vi "Returning A Value Complex Struct Added.vi"(8 "error in (no error)":errorcluster) -> ()   [LabVIEW 2009, in "LabVIEWWrapper_PassingDataSampleDLL.lvlib"]
doc: "int ReturningAValue_Integer (void);"
uses:
  LabVIEWWrapper_PassingDataSampleDLL.lvlib
  CustomControlsForStructs/ComplexStruct Polygon.ctl
  <vilib>/Utility/importsl/GetValueByPointer/GetValueByPointer.xnode
  <vilib>/Utility/importsl/GetValueByPointer/datatype.ctl
  PassingDataSampleDLL.dll
  Program Files (x86)/National Instruments/LabVIEW 2009/resource/lvimptsl.dll
panel:
  out "ComplexStruct Polygon":T1
  out "error out":errorcluster
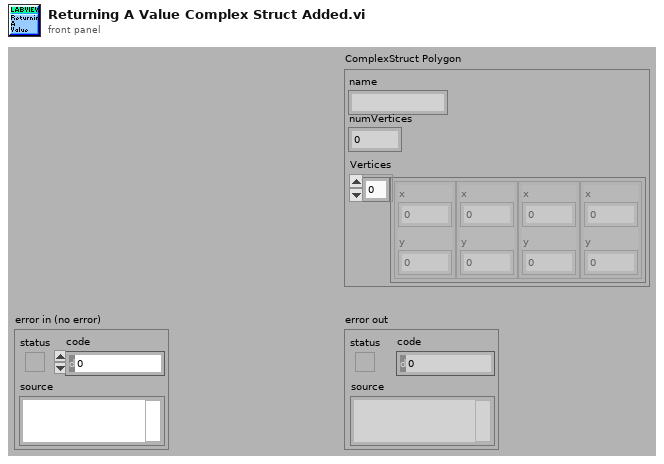
[diagram p1: front panel]
types:
  T1 = typedef "LabVIEWWrapper_PassingDataSampleDLL.lvlib/ComplexStruct Polygon.ctl" = cluster{"name":string, "numVertices":i32, "Vertices":cluster{"x":i32, "y":i32}[]}
  T2 = cluster{"Output":string, "Destination":i32, cluster{"Output":i32, "Output":i32}[]}
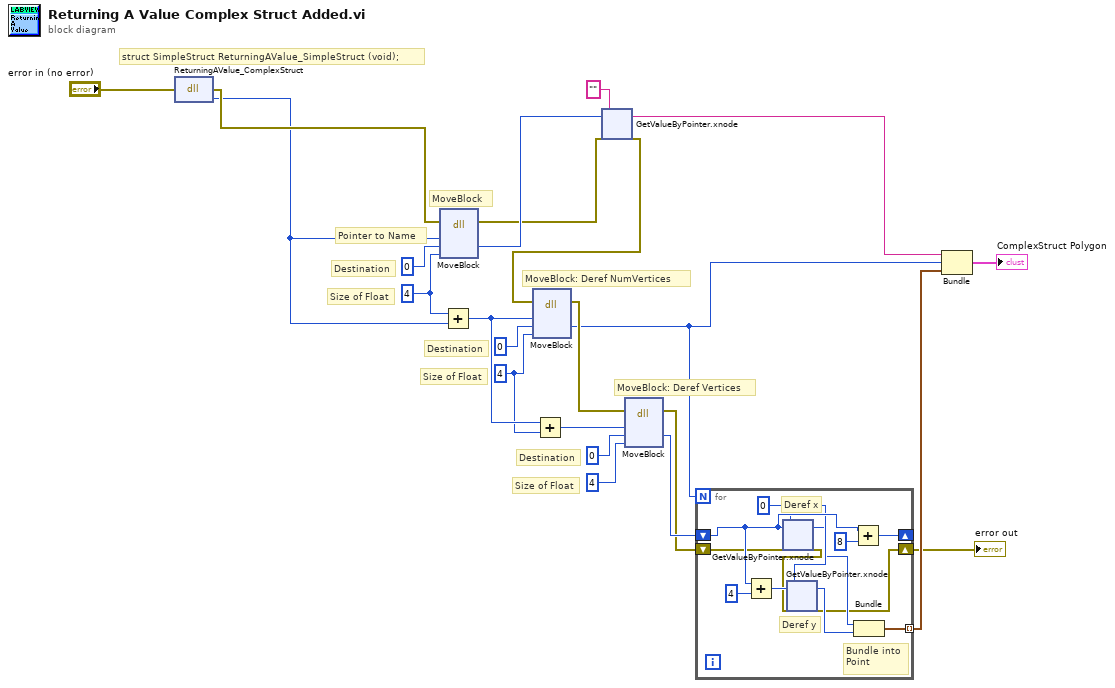
[diagram p0: block diagram]
diagram:
  w16 = 4 ("arg3")
  w14 = 4 ("arg3")
  # "Pointer to Name"
  # "Destination"
  # "Size of Float"
  # "MoveBlock: Deref Vertices"
  # "Destination"
  # "Size of Float"
  # "MoveBlock: Deref NumVertices"
  # "Destination"
  # "Size of Float"
  # "MoveBlock"
  # "struct SimpleStruct ReturningAValue_SimpleStruct (void);"
  n1 = dll-call lib="C:/My Dropbox/Systems Engineering Application/SDK/C Integration/LabVIEWWrapper/PassingDataSampleDLL.*" fn="ReturningAValue_ComplexStruct"(error in="error in (no error)") -> (error out=w8:errorcluster, "return type"=w7:i32)  [unwired: 2 in, 1 out]
  n2 = dll-call lib="LabVIEW" fn="MoveBlock"(error in=w8, "Address (Pointer)"=w7, "Destination"=0, "Size"=w14) -> (error out=w10:errorcluster, "Destination"=w12:i32)  [unwired: 5 in, 1 out]
  n3 = Add(x=w14, y=w7) -> (x+y=w17:i32)
  n4 = Add(x=w17, y=w16) -> (x+y=w18:i32)
  n5 = xnode "GetValueByPointer.xnode"("Pointer"=w12, "InputType"="", "ErrorIn"=w10) -> ("Output"=w5:string, "ErrorOut"=w9:errorcluster)  [unwired: 1 in]
  n6 = dll-call lib="LabVIEW" fn="MoveBlock"(error in=w9, "Address (Pointer)"=w17, "Destination"=0, "Size"=w16) -> (error out=w11:errorcluster, "Destination"=w4:i32)  [unwired: 5 in, 1 out]
  n7 = dll-call lib="LabVIEW" fn="MoveBlock"(error in=w11, "Address (Pointer)"=w18, "Destination"=0, "Size"=4 ("arg3")) -> (error out=w2:errorcluster, "Destination"=w15:i32)  [unwired: 5 in, 1 out]
  n8 = for {
    N: w4 -> [_]
    shift-right: [w31] -> _
    shift-left: w15 -> [w32]
    tunnel: [w27] -> w3 mode=indexing
    shift-right: [w24] -> w1
    shift-left: w2 -> [w26]
    w30 = 0
    # "Deref y"
    # "Deref x"
    # "Bundle into\nPoint"
    n9 = Add(x=w32, y=4) -> (x+y=w35:i32)
    n10 = xnode "GetValueByPointer.xnode"("Pointer"=w32, "InputType"=w30, "ErrorIn"=w26) -> ("Output"=w29:i32, "ErrorOut"=w25:errorcluster)  [unwired: 1 in]
    n11 = xnode "GetValueByPointer.xnode"("Pointer"=w35, "InputType"=w30, "ErrorIn"=w25) -> ("Output"=w28:i32, "ErrorOut"=w24:errorcluster)  [unwired: 1 in]
    n12 = Add(x=w32, y=8) -> (x+y=w31:i32)
    n13 = Bundle("Output"=w29, "Output"=w28) -> (w27:cluster{"Output":i32, "Output":i32})  [unwired: 1 in]
  }
  "error out" <- w1
  n14 = Bundle("Output"=w5, "Destination"=w4, w3) -> (→"ComplexStruct Polygon":T2)  [unwired: 1 in]
